vi "Read_Endpoint_State.vi"(0 "error in":errorcluster, 2 "Side":T3, 3 "node":string) -> (1 "error out":errorcluster, 4 "Endpoint State":T2)   [LabVIEW 2015]
doc: "Reads in the end point state"
uses:
  ROS/Code/SubVIs/BaxterSide.ctl
  ROS/Code/Console/Servers/ServerSubs/TopicDef.ctl
  ROS/Code/SubVIs/_ROSDirection.ctl
panel:
  out "Orientation":T1
  out "Reply":string
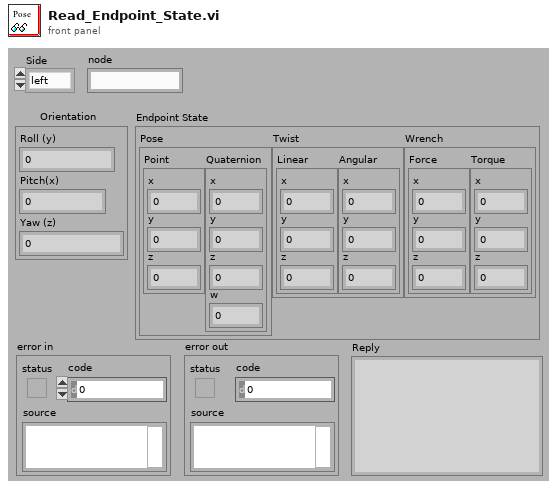
[diagram p1: front panel]
types:
  T1 = cluster{"Roll (y)":dbl, "Pitch(x)":dbl, "Yaw (z)":dbl}
  T2 = cluster{"Pose":cluster{"Point":cluster{"x":dbl, "y":dbl, "z":dbl}, "Quaternion":cluster{"x":dbl, "y":dbl, "z":dbl, "w":dbl}}, "Twist":cluster{"Linear":cluster{"x":dbl, "y":dbl, "z":dbl}, "Angular":cluster{"x":dbl, "y":dbl, "z":dbl}}, "Wrench":cluster{"Force":cluster{"x":dbl, "y":dbl, "z":dbl}, "Torque":cluster{"x":dbl, "y":dbl, "z":dbl}}}
  T3 = typedef "BaxterSide.ctl" = enum16{"left", "right"}
  T4 = typedef "TopicDef.ctl" = cluster{"Topic":string, "Type":string, "Action":T5, "Update (ms)":u16, "queue size":u16}
  T5 = typedef "_ROSDirection.ctl" = enum16{"Node", "Publisher", "Subscriber", "ServiceClient", "ServiceProvider"}
  T6 = typedef "_ROSControl.ctl" = cluster{"topic port":u16, "Node":string, "topic":string, "type":string, "node port":u16, "error ":errorcluster, "Direction":T5, "Update (ms)":u16, "FIFO size":u16}
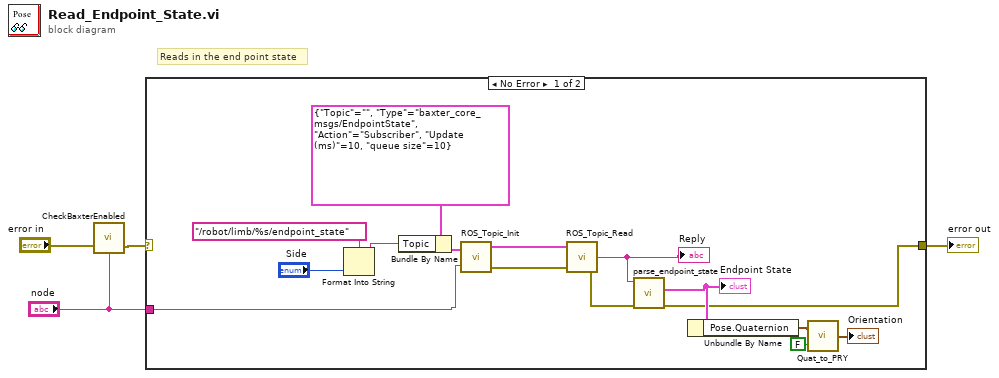
[diagram p0: block diagram]
diagram:
  # "Reads in the end point state"
  n1 = call "CheckBaxterEnabled.vi"("error in"="error in", "node"="node") -> ("error out"=w3:errorcluster)  [unwired: 2 in]
  n2 = case shown="No Error" w3 {
    selector: w3 -> [_ w20]
    tunnel: [w5 w20] -> w4
    tunnel: "node" -> [w8 _]
    frame No Error {
      n3 = Format Into String(format string="/robot/limb/%s/endpoint_state" ("topic"), "Side") -> (resulting string=w11:string)  [unwired: 2 in, 1 out]
      n4 = Bundle By Name(cluster=T4 {"Topic"="", "Type"="baxter_core_msgs/EndpointState", "Action"=enum."Subscriber", "Update (ms)"=10, "queue size"=10} ("Definitions"), "Topic"=w11) -> (w9:T4)
      n5 = call "ROS_Topic_Init.vi"("Definitions"=w9, "node"=w8) -> ("ROS out"=w19:T6, "error out"=w7:errorcluster)  [unwired: 1 in]
      n6 = call "ROS_Topic_Read.vi"("error in (no error)"=w7, "ROS in"=w19) -> ("error out"=w6:errorcluster, "Reply"=w18:string)  [unwired: 1 in, 1 out]
      "Reply" <- w18
      n7 = call "parse_endpoint_state.vi"("error in"=w6, "msg in"=w18) -> ("error out"=w5:errorcluster, "Endpoint State"=w17:T2)  [unwired: 3 in, 1 out]
      "Endpoint State" <- w17
      n8 = Unbundle By Name(w17) -> ("Pose.Quaternion"=w16:cluster{"x":dbl, "y":dbl, "z":dbl, "w":dbl})
      n9 = call "Quat_to_PRY.vi"("toDegrees? (T)"=FALSE, "Quaternion"=w16) -> ("Orientation"=→"Orientation":T1)
    }
    frame Error {
    }
  }
  "error out" <- w4
